vi "Inspect Fiducials.vi"(7 "Console Log in":refnum<class "Console Log.lvclass">, 8 "error in":errorcluster, 11 "Gluing Procedure in":refnum<class "Gluing Procedure.lvclass">) -> (0 "error out":errorcluster, 1 "Step canceled?":bool, 3 "Gluing Procedure out":refnum<class "Gluing Procedure.lvclass">, 5 "Console Log out":refnum<class "Console Log.lvclass">)   [LabVIEW 2017, in "Gluing Procedure.lvclass"]
uses:
  Gluing Procedure.lvclass
  Shared Components/CameraTool Class/CameraTool Class.lvclass
  Shared Components/Vec3d Class/Vec3d Class.lvclass
  <vilib>/vision/Image Controls.llb/IMAQ Image.ctl
  Shared Components/Utils/Type Definitions/Physical Image.ctl
  Shared Components/Utils/Type Definitions/Fiducial with Source.ctl
  Shared Components/Utils/Type Definitions/Fiducial Image.ctl
  Shared Components/Utils/Type Definitions/Part Fiducials.ctl
  Type Definitions/Inspect Fuducials.ctl
  Shared Components/Gantry Class/Gantry Class.lvclass
  Shared Components/FlexWorktable/FlexWorktable.lvclass
  Application Utilities/Console Log/Console Log.lvclass
panel:
  # "This VI needs to load the camera and inspect fiducials\nfor selected chuck/slots for HDIs, Stamps, Weights, and BBMs\n\nTo think about:\nShould split up HDI, Stamp, Weight, and BBMs into their own sub VIs, where this one calls them?"
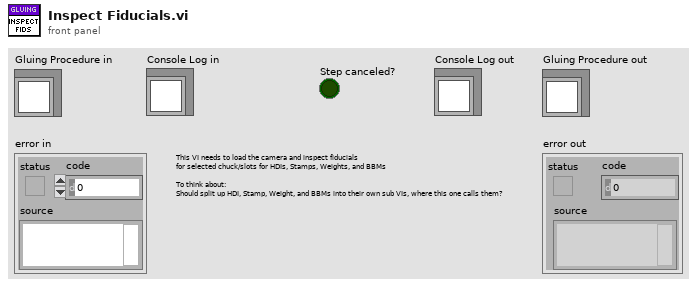
[diagram p1: front panel]
types:
  T1 = typedef "Inspect Fuducials.ctl" = cluster{"Path Fiducials":cluster{"HDI Fiducials":T2, "Stamp Fiducials":T2, "Weight Fiducials":T2, "BBM Fiducials":T2}[], "Has been run?":bool}
  T2 = typedef "Part Fiducials.ctl" = cluster{"Fiducials":T3[], "Chuck":i32, "Slot":i32}
  T3 = typedef "Fiducial Image.ctl" = cluster{"Fiducial Image":T4, "Selected Fiducial":T6, "fiducial name":string}
  T4 = typedef "Physical Image.ctl" = cluster{"Image Position":refnum<class "Vec3d Class.lvclass">, "Image Reference":T5, "Field of View":cluster{"x(mm)":dbl, "y(mm)":dbl}}
  T5 = typedef "IMAQ Image.ctl" = refnum<image>
  T6 = typedef "Fiducial with Source.ctl" = cluster{"Fiducial Image Coordinate":refnum<class "Vec3d Class.lvclass">, "Fiducial Source":enum16{"Pattern Recognition", "User", "Error", "Default"}}
  T7 = cluster{"HDI Fiducials":T2, "Stamp Fiducials":T2, "Weight Fiducials":T2, "BBM Fiducials":T2}
  T8 = typedef "Configure.ctl" = cluster{"Has been run?":bool, "Active Paths":T9, "Glue Pathways":T10, "Chuck Module Used for BBM:":T12}
  T9 = typedef "Active Paths.ctl" = bool[]
  T10 = typedef "Glue Paths.ctl" = T11[]
  T11 = typedef "Glue Path.ctl" = cluster{"HDI Slot ":i32, "Stamp Slot":i32, "Glue Slot":i32, "Weight Slot":i32, "BBM Slot":i32}
  T12 = typedef "BBM Chuck Used.ctl" = i32
  T13 = cluster{"HDI Fiducials":T2, "Stamp Fiducials":T2, "Weight Fiducials":T2, "BBM Fiducials":T2}[]
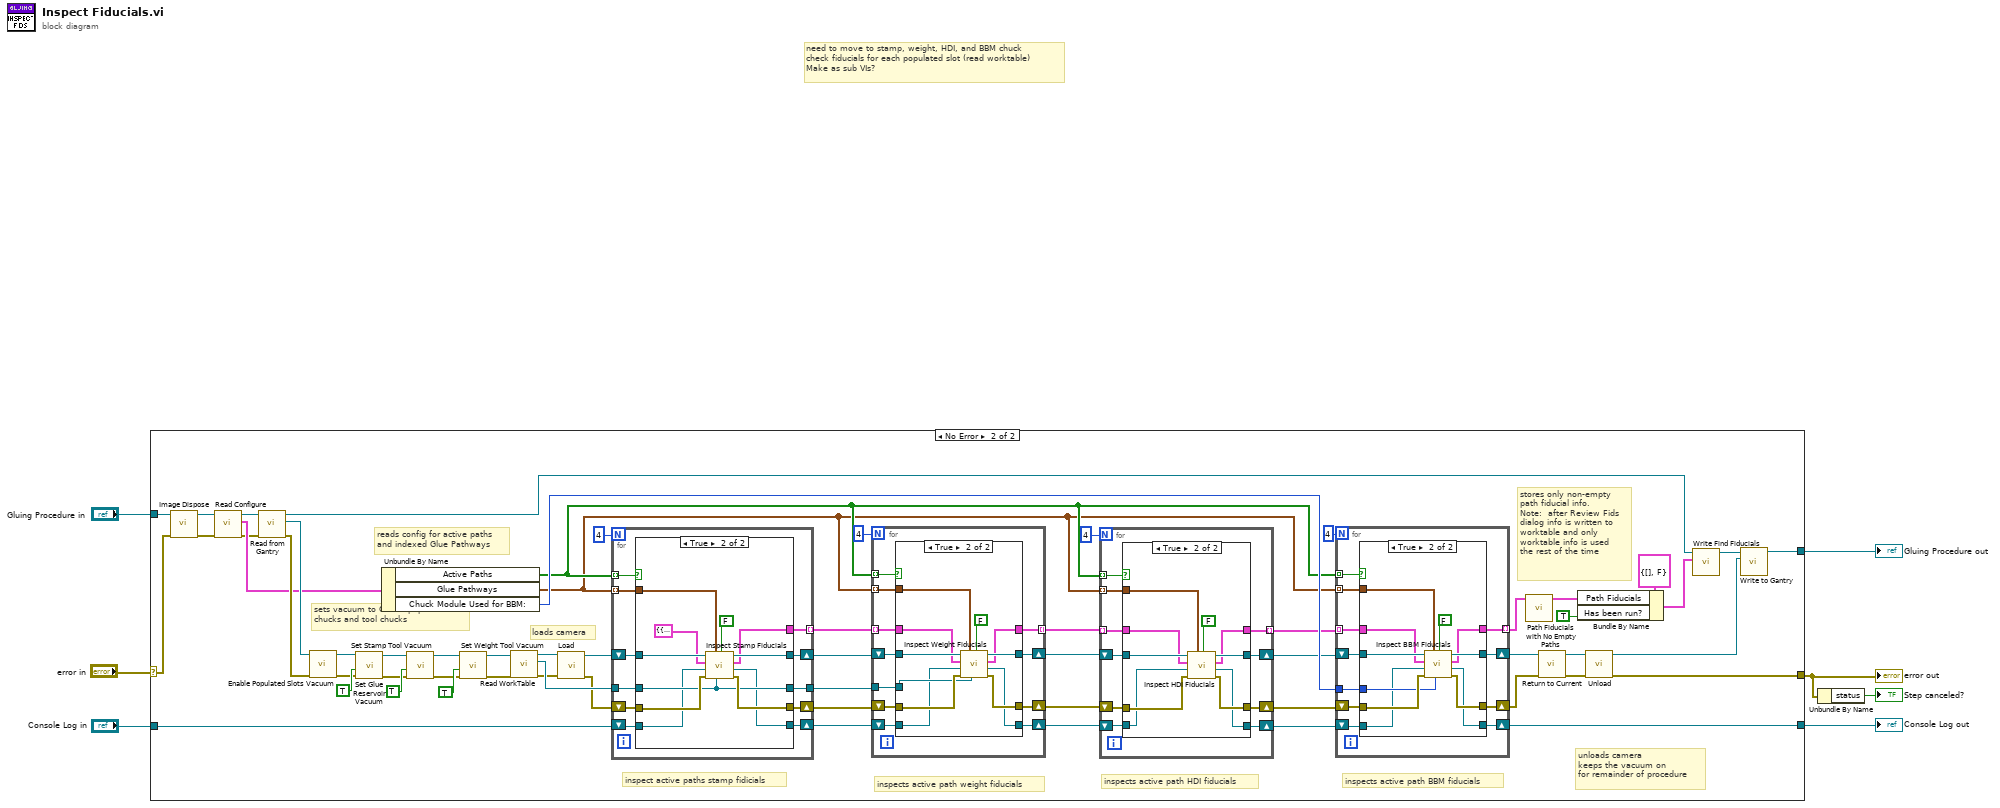
[diagram p0: block diagram]
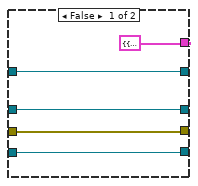
[diagram p6: hidden frame]
diagram:
  # "need to move to stamp, weight, HDI, and BBM chuck\ncheck fiducials for each populated slot (read worktable)\nMake as sub VIs?"
  n1 = case shown="No Error" "error in" {
    selector: "error in" -> [w9 w70]
    tunnel: "Gluing Procedure in" -> [w10 w71]
    tunnel: [w10 w34] -> w5
    tunnel: [w9 w22] -> w3
    tunnel: [w8 w13] -> w4
    tunnel: "Console Log in" -> [w8 w17]
    frame Error {
    }
    frame No Error {
      # "stores only non-empty\npath fiducial info.\nNote:  after Review Fids\ndialog info is written to \nworktable and only \nworktable info is used\nthe rest of the time"
      # "loads camera"
      # "unloads camera\nkeeps the vacuum on\nfor remainder of procedure"
      # "inspects active path BBM fiducials"
      # "inspects active path HDI fiducials"
      # "reads config for active paths\nand indexed Glue Pathways"
      # "inspects active path weight fiducials"
      # "inspect active paths stamp fidicials"
      # "sets vacuum to ON for populated\nchucks and tool chucks"
      n2 = call "Image Dispose.vi"("error in"=w70, "Gluing Procedure in"=w71) -> ("error out"=w33:errorcluster, "Gluing Procedure out"=w57:refnum<class "Gluing Procedure.lvclass">)  [unwired: 8 in]
      n3 = call "Read Configure.vi"("error in (no error)"=w33, "Gluing Procedure in"=w57) -> ("error out"=w32:errorcluster, "Configure"=w55:T8, "Gluing Procedure out"=w56:refnum<class "Gluing Procedure.lvclass">)  [unwired: 7 in]
      n4 = call "Read from Gantry.vi"("error in (no error)"=w32, "Gluing Procedure in"=w56) -> ("error out"=w68:errorcluster, "Gantry"=w69:refnum<class "Gantry Class.lvclass">, "Gluing Procedure out"=w25:refnum<class "Gluing Procedure.lvclass">)  [unwired: 7 in]
      n5 = call-dynamic "Enable Populated Slots Vacuum.vi"("error in"=w68, "Gantry in"=w69) -> ("error out"=w31:errorcluster, "Gantry out"=w65:refnum<class "Gantry Class.lvclass">)  [unwired: 8 in]
      n6 = call-dynamic "Set Glue Reservoir Vacuum.vi"("error in (no error)"=w31, "On/Off"=TRUE, "Gantry Class in"=w65) -> ("error out"=w30:errorcluster, "Gantry Class out"=w63:refnum<class "Gantry Class.lvclass">)  [unwired: 7 in]
      n7 = Unbundle By Name(w55) -> ("Active Paths"=w43:T9, "Glue Pathways"=w42:T10, "Chuck Module Used for BBM:"=w47:T12)
      n8 = call-dynamic "Set Stamp Tool Vacuum.vi"("error in"=w30, "On/Off"=TRUE, "Gantry in"=w63) -> ("error out"=w29:errorcluster, "Gantry out"=w61:refnum<class "Gantry Class.lvclass">)  [unwired: 7 in]
      n9 = call-dynamic "Set Weight Tool Vacuum.vi"("error in"=w29, "On/Off"=TRUE, "Gantry in"=w61) -> ("error out"=w28:errorcluster, "Gantry out"=w59:refnum<class "Gantry Class.lvclass">)  [unwired: 7 in]
      n10 = call-dynamic "Read WorkTable.vi"("error in"=w28, "Gantry Class in"=w59) -> ("error out"=w27:errorcluster, "Worktable"=w58:refnum<class "FlexWorktable.lvclass">, "Gantry Class out"=w67:refnum<class "Gantry Class.lvclass">)  [unwired: 7 in]
      n11 = call "Load.vi"("error in"=w27, "Gantry In"=w67) -> ("error out"=w52:errorcluster, "CameraTool out"=w66:refnum<class "CameraTool Class.lvclass">)  [unwired: 8 in]
      n12 = for {
        N: 4 -> [_]
        tunnel: w58 -> [w157]
        tunnel: w43 -> [w156] mode=indexing
        shift-right: [w153] -> w50
        shift-left: w66 -> [w158]
        tunnel: w42 -> [w155] mode=indexing
        tunnel: [w154] -> w51 mode=indexing
        shift-right: [w151] -> w49
        shift-left: w52 -> [w152]
        tunnel: [w150] -> w48
        shift-right: [w148] -> w16
        shift-left: w17 -> [w149]
        n13 = case shown="True" w156 {
          tunnel: w158 -> [w163 w174]
          tunnel: w157 -> [w162 w169]
          tunnel: w155 -> [_ w173]
          tunnel: [T7 {"HDI Fiducials"={"Fiducials"=[], "Chuck"=0, "Slot"=0}, "Stamp Fiducials"={"Fiducials"=[], "Chuck"=0, "Slot"=0}, "Weight Fiducials"={"Fiducials"=[], "Chuck"=0, "Slot"=0}, "BBM Fiducials"={"Fiducials"=[], "Chuck"=0, "Slot"=0}} ("Single Path in") w167] -> w154
          tunnel: [w163 w168] -> w153
          tunnel: w152 -> [w161 w171]
          tunnel: [w161 w170] -> w151
          tunnel: [w162 w169] -> w150
          tunnel: w149 -> [w159 w165]
          tunnel: [w159 w164] -> w148
          frame False {
          }
          frame True {
            n14 = call "Inspect Stamp Fiducials.vi"("Dispose Images?"=FALSE, "WorkTable Class in"=w169, "Glue Pathways"=w173, "error in"=w171, "Console Log in"=w165, "Single Path in"=T7 {"HDI Fiducials"={"Fiducials"=[], "Chuck"=0, "Slot"=0}, "Stamp Fiducials"={"Fiducials"=[], "Chuck"=0, "Slot"=0}, "Weight Fiducials"={"Fiducials"=[], "Chuck"=0, "Slot"=0}, "BBM Fiducials"={"Fiducials"=[], "Chuck"=0, "Slot"=0}}, "CameraTool in"=w174) -> ("error out"=w170:errorcluster, "Console Log out"=w164:refnum<class "Console Log.lvclass">, "Single Path out"=w167:T7, "CameraTool out"=w168:refnum<class "CameraTool Class.lvclass">)  [unwired: 1 in]
          }
        }
      }
      n15 = for {
        N: 4 -> [_]
        tunnel: w48 -> [w131]
        tunnel: w43 -> [w130] mode=indexing
        shift-right: [w126] -> w45
        shift-left: w50 -> [w132]
        tunnel: w51 -> [w129] mode=indexing
        tunnel: w42 -> [w128] mode=indexing
        tunnel: [w127] -> w46 mode=indexing
        shift-right: [w124] -> w44
        shift-left: w49 -> [w125]
        shift-right: [w122] -> w15
        shift-left: w16 -> [w123]
        n16 = case shown="True" w130 {
          tunnel: w132 -> [w135 w142]
          tunnel: w131 -> [_ w139]
          tunnel: w129 -> [w136 w141]
          tunnel: w128 -> [_ w147]
          tunnel: [w136 w140] -> w127
          tunnel: [w135 w145] -> w126
          tunnel: w125 -> [w134 w143]
          tunnel: [w134 w144] -> w124
          tunnel: w123 -> [w133 w138]
          tunnel: [w133 w137] -> w122
          frame False {
          }
          frame True {
            n17 = call "Inspect Weight Fiducials.vi"("Dispose Images?"=FALSE, "WorkTable Class in"=w139, "Glue Pathways"=w147, "error in"=w143, "Console Log in"=w138, "Single Path in"=w141, "CameraTool in"=w142) -> ("error out"=w144:errorcluster, "Console Log out"=w137:refnum<class "Console Log.lvclass">, "Single Path out"=w140:T7, "CameraTool out"=w145:refnum<class "CameraTool Class.lvclass">)  [unwired: 1 in]
          }
        }
      }
      n18 = for {
        N: 4 -> [_]
        tunnel: w43 -> [w80] mode=indexing
        shift-right: [w76] -> w40
        shift-left: w45 -> [w81]
        tunnel: w46 -> [w79] mode=indexing
        tunnel: w42 -> [w78] mode=indexing
        tunnel: [w77] -> w41 mode=indexing
        shift-right: [w74] -> w39
        shift-left: w44 -> [w75]
        shift-right: [w72] -> w14
        shift-left: w15 -> [w73]
        n19 = case shown="True" w80 {
          tunnel: w81 -> [w84 w90]
          tunnel: w79 -> [w85 w89]
          tunnel: w78 -> [_ w95]
          tunnel: [w85 w88] -> w77
          tunnel: [w84 w93] -> w76
          tunnel: w75 -> [w83 w91]
          tunnel: [w83 w92] -> w74
          tunnel: w73 -> [w82 w87]
          tunnel: [w82 w86] -> w72
          frame False {
          }
          frame True {
            n20 = call "Inspect HDI Fiducials.vi"("Dispose Images?"=FALSE, "Glue Pathways"=w95, "error in"=w91, "Console Log in"=w87, "Single Path in"=w89, "CameraTool in"=w90) -> ("error out"=w92:errorcluster, "Console Log out"=w86:refnum<class "Console Log.lvclass">, "Single Path out"=w88:T7, "CameraTool out"=w93:refnum<class "CameraTool Class.lvclass">)  [unwired: 2 in]
          }
        }
      }
      n21 = for {
        N: 4 -> [_]
        tunnel: w43 -> [w105] mode=indexing
        shift-right: [w101] -> w38
        shift-left: w40 -> [w106]
        tunnel: w41 -> [w104] mode=indexing
        tunnel: w42 -> [w103] mode=indexing
        tunnel: [w102] -> w11 mode=indexing
        shift-right: [w99] -> w36
        shift-left: w39 -> [w100]
        tunnel: w47 -> [w98]
        shift-right: [w96] -> w13
        shift-left: w14 -> [w97]
        n22 = case shown="True" w105 {
          tunnel: w106 -> [w109 w116]
          tunnel: w104 -> [w110 w114]
          tunnel: w103 -> [_ w121]
          tunnel: [w110 w115] -> w102
          tunnel: [w109 w119] -> w101
          tunnel: w100 -> [w108 w117]
          tunnel: [w108 w118] -> w99
          tunnel: w98 -> [_ w113]
          tunnel: w97 -> [w107 w112]
          tunnel: [w107 w111] -> w96
          frame False {
          }
          frame True {
            n23 = call "Inspect BBM Fiducials.vi"("Dispose Images?"=FALSE, "BBM Chuck"=w113, "Glue Pathways"=w121, "error in"=w117, "Console Log in"=w112, "Single Path in"=w114, "CameraTool in"=w116) -> ("error out"=w118:errorcluster, "Console Log out"=w111:refnum<class "Console Log.lvclass">, "Single Path out"=w115:T7, "CameraTool out"=w119:refnum<class "CameraTool Class.lvclass">)  [unwired: 1 in]
          }
        }
      }
      n24 = call "Path Fiducials with No Empty Paths.vi"("Path Fiducials"=w11) -> ("Path Fiducials (no empty paths)"=w12:T13)  [unwired: 10 in]
      n25 = call-dynamic "Return to Current.vi"("error in"=w36, "Gantry in"=w38) -> ("error out"=w35:errorcluster, "Gantry out"=w37:refnum<class "CameraTool Class.lvclass">)  [unwired: 8 in]
      n26 = Bundle By Name(cluster=T1 {"Path Fiducials"=[], "Has been run?"=FALSE} ("Find Fiducials"), "Path Fiducials"=w12, "Has been run?"=TRUE) -> (w26:T1)
      n27 = call "Unload.vi"("error in"=w35, "CameraTool in"=w37) -> ("error out"=w22:errorcluster, "Gantry out"=w23:refnum<class "Gantry Class.lvclass">)  [unwired: 8 in]
      n28 = call "Write Find Fiducials.vi"("Find Fiducials"=w26, "Gluing Procedure in"=w25) -> ("Gluing Procedure out"=w24:refnum<class "Gluing Procedure.lvclass">)  [unwired: 8 in, 1 out]
      n29 = call "Write to Gantry.vi"("Gantry"=w23, "Gluing Procedure in"=w24) -> ("Gluing Procedure out"=w34:refnum<class "Gluing Procedure.lvclass">)  [unwired: 8 in, 1 out]
    }
  }
  "error out" <- w3
  "Gluing Procedure out" <- w5
  "Console Log out" <- w4
  n30 = Unbundle By Name(w3) -> ("status"=→"Step canceled?":bool)
